vi "COM_send_data.vi"(8 "data":u8[](array[numeric]), 10 "baud rate (9600)":u32=115200 caption="波特率(115200)", 11 "VISA name":refnum<visa-resource-name>) -> (3 "return":i32)   [LabVIEW 2016]
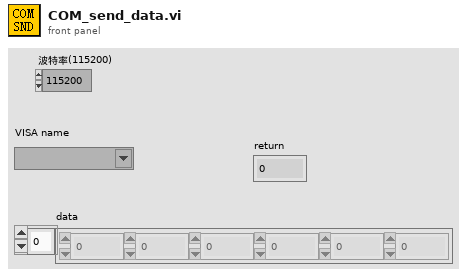
[diagram p1: front panel]
types:
  T1 = enum16{"initial", "write", "read", "release", "change"}
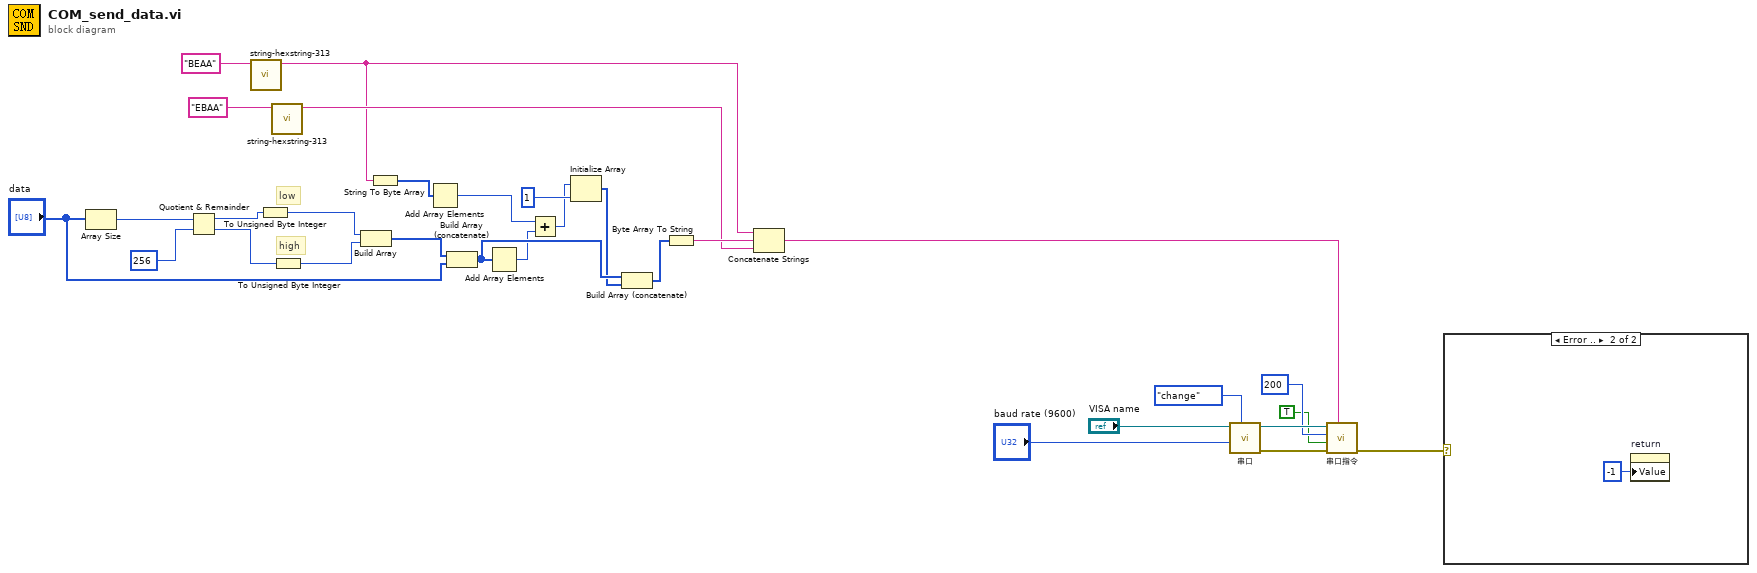
[diagram p0: block diagram]
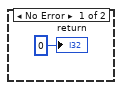
[diagram p2: hidden frame]
diagram:
  # "high"
  # "low"
  n1 = Array Size(array="data") -> (size(s)=w10:i32)
  n2 = Quotient & Remainder(x=w10, y=256) -> (x-y*floor(x/y)=w28:i32, floor(x/y)=w29:i32)
  n3 = call "string-hexstring-313.vi"("字符串"="BEAA") -> ("十六进制整型字符串"=w15:string)  [unwired: 10 in]
  n4 = To Unsigned Byte Integer(number=w28) -> (unsigned 8bit integer=w26:u8)
  n5 = call "string-hexstring-313.vi"("字符串"="EBAA") -> ("十六进制整型字符串"=w16:string)  [unwired: 10 in]
  n6 = To Unsigned Byte Integer(number=w29) -> (unsigned 8bit integer=w25:u8)
  n7 = Build Array(w26, w25) -> (w24:u8[])
  n8 = String To Byte Array(string=w15) -> (unsigned byte array=w14:u8[])
  n9 = Add Array Elements(numeric array=w14) -> (sum=w13:u8)
  n10 = Build Array (concatenate)(w24, "data") -> (w20:u8[])
  n11 = Add Array Elements(numeric array=w20) -> (sum=w12:u8)
  n12 = Add(x=w13, y=w12) -> (x+y=w11:u8)
  n13 = Initialize Array(w11, 1 ("dimension size")) -> (w19:u8[])
  n14 = Build Array (concatenate)(w20, w19) -> (w18:u8[])
  n15 = Byte Array To String(unsigned byte array=w18) -> (string=w22:string)
  n16 = Concatenate Strings(w15, w22, w16) -> (w4:string)
  n17 = call "串口.vi"("case"=T1."change", "baud rate (9600)"="baud rate (9600)", "VISA name"="VISA name") -> ("error out"=w3:errorcluster, "VISA resource name out"=w8:refnum<visa-resource-name>)  [unwired: 5 in, 2 out]
  n18 = call "串口指令.vi"("write buffer"=w4, "error in"=w3, "是否握手"=TRUE, "limit"=200, "VISA resource name"=w8) -> ("error out"=w2:errorcluster)  [unwired: 2 in, 4 out]
  n19 = case shown="Error .." w2 {
    frame No Error {
      "return" <- 0 ("return")
    }
    frame Error {
      n20 = property on="return" class="DigNum (strict)"("Value"=-1 ("return")) -> ()  [unwired: 2 in, 2 out]
    }
  }
